vi "Insight_Streaming_Example.vi"() -> ()   [LabVIEW 2011]
panel:
  out "error out":errorcluster
  out "size(s)":i32
  out "Waveform Chart":u16[](graph)
  in  "stop":bool
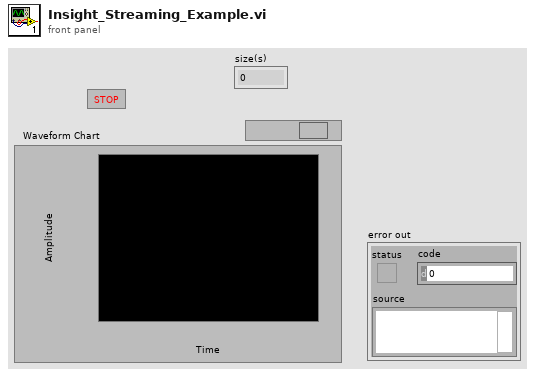
[diagram p1: front panel]
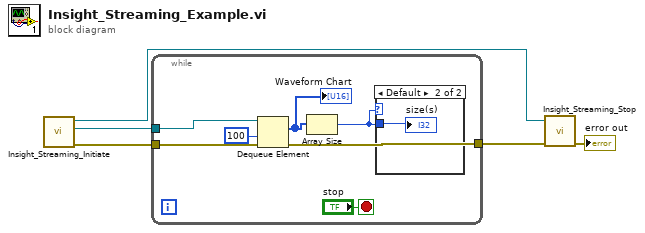
[diagram p0: block diagram]
diagram:
  n1 = call "Insight_Streaming_Initiate.vi"() -> ("error out"=w4:errorcluster, "Data Queue"=w5:refnum<queue>, "Streaming VI"=w2:refnum<vi>)  [unwired: 9 in]
  n2 = while {
    tunnel: w5 -> [w12]
    tunnel: w4 -> [w11]
    tunnel: [w9] -> w3
    stop <- "stop" stop-if-true
    n3 = Dequeue Element(queue=w12, timeout in ms (-1)=100, error in (no error)=w11) -> (element=w7:u16[], error out=w9:errorcluster)  [unwired: 2 out]
    "Waveform Chart" <- w7
    n4 = Array Size(array=w7) -> (size(s)=w6:i32)
    n5 = case shown="Default" w6 {
      tunnel: w6 -> [_ w13]
      frame 0 {
      }
      frame Default {
        "size(s)" <- w13
      }
    }
  }
  n6 = call "Insight_Streaming_Stop.vi"("error in (no error)"=w3, "Streaming VI"=w2) -> ("error out"=→"error out":errorcluster)  [unwired: 9 in]
